vi "terminate.vi"(8 "error in (no error)":errorcluster, 11 "GenericPlugin in":refnum<class "SignalWriterMH110203USBStepperMotor.lvclass">) -> (0 "error out":errorcluster, 3 "GenericPlugin out":refnum<class "SignalWriterMH110203USBStepperMotor.lvclass">)   [LabVIEW 2010, in "SignalWriterMH110203USBStepperMotor.lvclass"]
doc: "The dynamic dispatch version of this VI terminates the plug-in object by releasing all of its resources."
uses:
  SignalWriterMH110203USBStepperMotor.lvclass
  GenericSignalWriter/GenericSignalWriter/GenericSignalWriter.lvclass
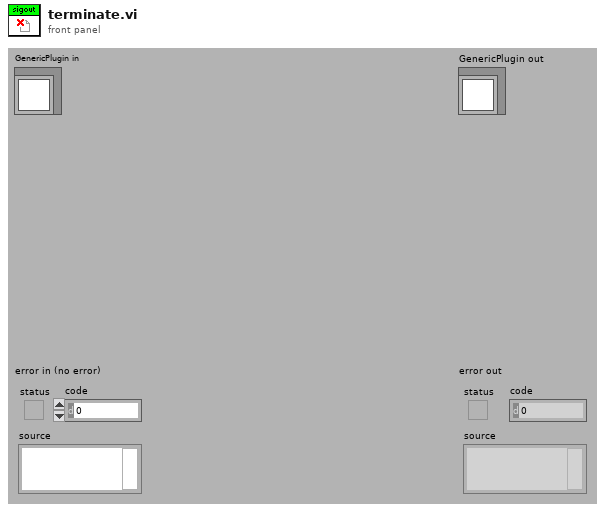
[diagram p1: front panel]
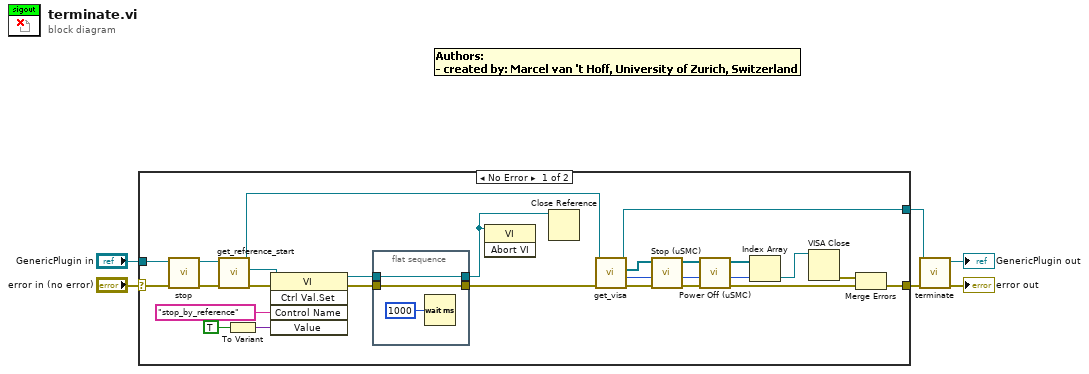
[diagram p0: block diagram]
diagram:
  n1 = case shown="No Error" "error in (no error)" {
    selector: "error in (no error)" -> [w17 w36]
    tunnel: [w29 w36] -> w3
    tunnel: "GenericPlugin in" -> [w19 w35]
    tunnel: [w28 w35] -> w2
    frame No Error {
      n2 = call-dynamic "stop.vi"("error in (no error)"=w17, "WriteSignalsGenericPlugin in"=w19) -> ("error out"=w16:errorcluster, "WriteSignalsGenericPlugin out"=w18:refnum<class "SignalWriterMH110203USBStepperMotor.lvclass">)  [unwired: 8 in]
      n3 = call-dynamic "get_reference_start.vi"("error in (no error)"=w16, "SignalWriterMH110203USBStepperMotor in"=w18) -> ("error out"=w22:errorcluster, "vi reference"=w20:refnum<vi>, "SignalWriterMH110203USBStepperMotor out"=w21:refnum<class "SignalWriterMH110203USBStepperMotor.lvclass">)  [unwired: 7 in]
      n4 = To Variant(anything=TRUE) -> (Variant=w25:variant)
      n5 = invoke class="VI" method="Ctrl Val.Set"(reference=w20, error in=w22, "Control Name"="stop_by_reference", "Value"=w25) -> (reference out=w15:refnum<vi>, error out=w14:errorcluster)  [unwired: 1 in, 3 out]
      n6 = flat-sequence {
        tunnel: [w33] -> w13
        tunnel: w15 -> [w33]
        tunnel: [w32] -> w12
        tunnel: w14 -> [w32]
        frame #0 {
          n7 = Wait (ms)(milliseconds to wait=u32 1000) -> ()  [unwired: 1 out]
        }
      }
      n8 = invoke class="VI" method="Abort VI"(reference=w13) -> ()  [unwired: 2 in, 3 out]
      n9 = Close Reference(reference=w13) -> ()  [unwired: 1 in, 1 out]
      n10 = call-dynamic "get_visa.vi"("error in (no error)"=w12, "SignalWriterMH110203USBStepperMotor in"=w21) -> ("error out"=w26:errorcluster, "axis"=w8:i32, "visa array"=w27:refnum<visa-resource-name>[], "SignalWriterMH110203USBStepperMotor out"=w28:refnum<class "SignalWriterMH110203USBStepperMotor.lvclass">)  [unwired: 6 in]
      n11 = call "Stop (uSMC).vi"("error in (no error)"=w26, "Index"=w8, "Visa array in"=w27) -> ("error out"=w11:errorcluster, "Visa array out"=w10:refnum<visa-resource-name>[])  [unwired: 7 in]
      n12 = call "Power Off (uSMC).vi"("error in (no error)"=w11, "Index"=w8, "Visa Array in"=w10) -> ("error out"=w31:errorcluster, "Visa Array out"=w9:refnum<visa-resource-name>[])  [unwired: 7 in]
      n13 = Index Array(array=w9, index=w8) -> (element=w7:refnum<visa-resource-name>)
      n14 = VISA Close(VISA resource name=w7) -> (error out=w30:errorcluster)  [unwired: 1 in]
      n15 = Merge Errors(w30, w31) -> (w29:errorcluster)
    }
    frame Error {
    }
  }
  n16 = call-parent "terminate.vi"("error in (no error)"=w3, "GenericPlugin in"=w2) -> ("error out"=→"error out":errorcluster, "GenericPlugin out"=→"GenericPlugin out":refnum<class "SignalWriterMH110203USBStepperMotor.lvclass">)  [unwired: 8 in]
